vi "Poll Event.vi"(8 "error in":errorcluster) -> (0 "error out":errorcluster, 1 "Event Data":u8[](array[numeric]), 2 "Event Type":u32 format="%.0x", 3 "Return":i32)   [LabVIEW 2015, in "LibSDL2.lvlib"]
doc: "Polls for currently pending events.\n\nIf event is not NULL, the next event is removed from the queue and stored in the SDL_Event structure pointed to by event.\n\nAs this function implicitly calls SDL_PumpEvents, you can only call this function in the thread that set the video mode.\n\nReturns 1 if there are any pending events, or 0 if there are none available."
uses:
  LibSDL2.lvlib
  DLL/SDL2.dll
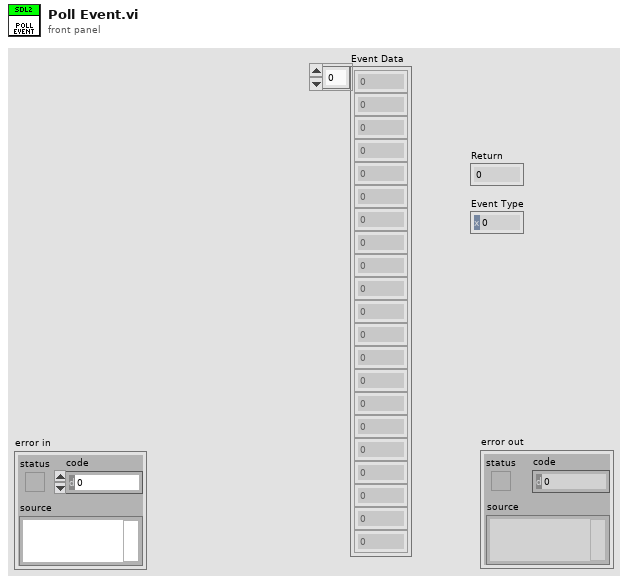
[diagram p1: front panel]
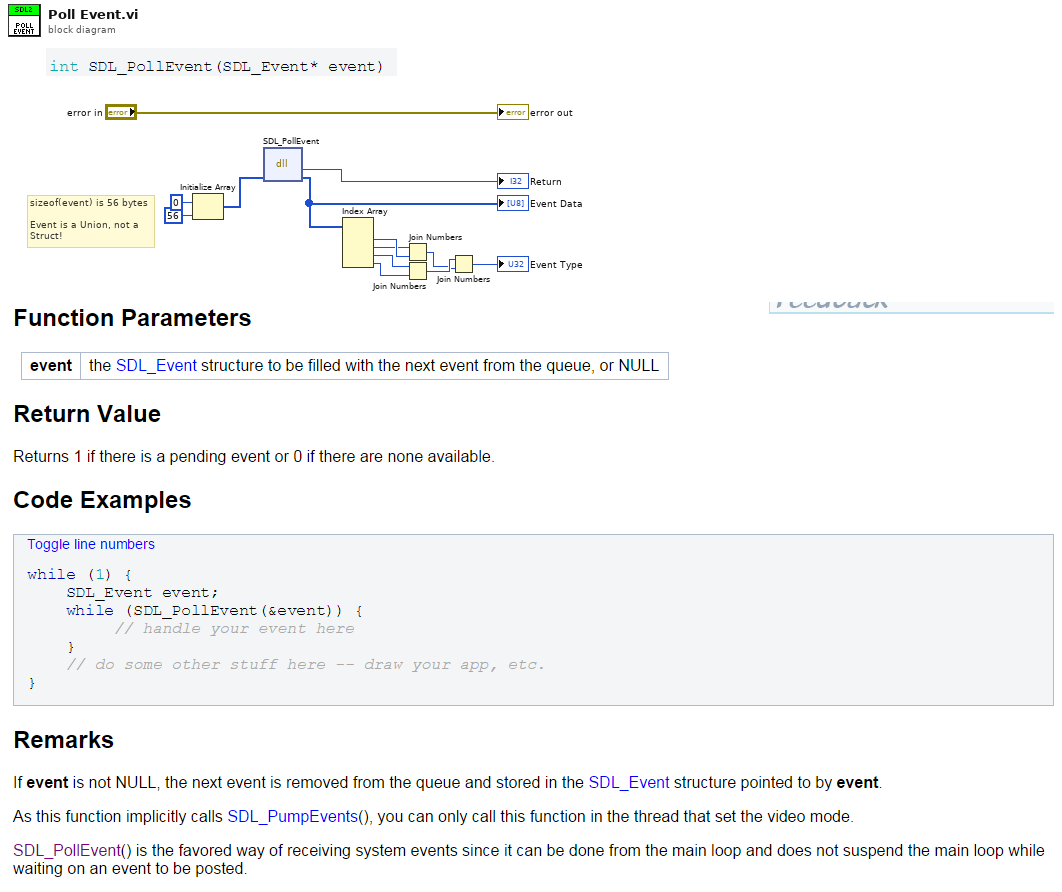
[diagram p0: block diagram]
diagram:
  # "sizeof(event) is 56 bytes\n\nEvent is a Union, not a Struct!"
  n1 = Initialize Array(u8 0, 56 ("dimension size")) -> (w10:u8[])
  n2 = dll-call lib="C:/dev/PGS/LabSDL2/Source/Libraries/LibSDL2 Wrapper/DLL/SDL2.dll" fn="SDL_PollEvent"("event"=w10) -> ("return type"=→"Return":i32, "event"=w9:u8[])  [unwired: 3 in, 2 out]
  "Event Data" <- w9
  n3 = Index Array(array=w9) -> (element #1=w8:u8, element #2=w7:u8, element #3=w6:u8, element #4=w5:u8)  [unwired: 4 in]
  n4 = Join Numbers(hi=w7, lo=w8) -> ((hi.lo)=w3:u16)
  n5 = Join Numbers(hi=w6, lo=w5) -> ((hi.lo)=w4:u16)
  n6 = Join Numbers(hi=w4, lo=w3) -> ((hi.lo)=→"Event Type":u32)
  "error out" <- "error in"
